vi "Set Cluster Values from JSON String Poly.vi"   [LabVIEW 2023]
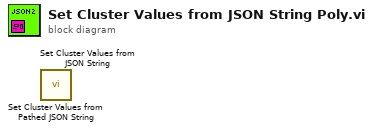
[diagram p0: block diagram]
diagram:
  n1 = call "Set Cluster Values from Pathed JSON String.vi"() -> ()  [unwired: 11 in, 1 out]
  n2 = call "Set Cluster Values from JSON String.vi"() -> ()  [unwired: 11 in, 1 out]
